vi "path_test.vi"() -> ()   [LabVIEW 2011]
panel:
  out "String":string
  out "size(s)":i32
  out "output string":string
  out "relative":bool
  out "array of strings":string[](array[string])
  in  "path 2":path
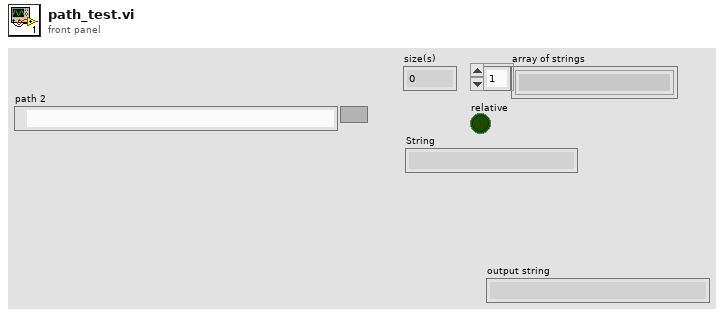
[diagram p1: front panel]
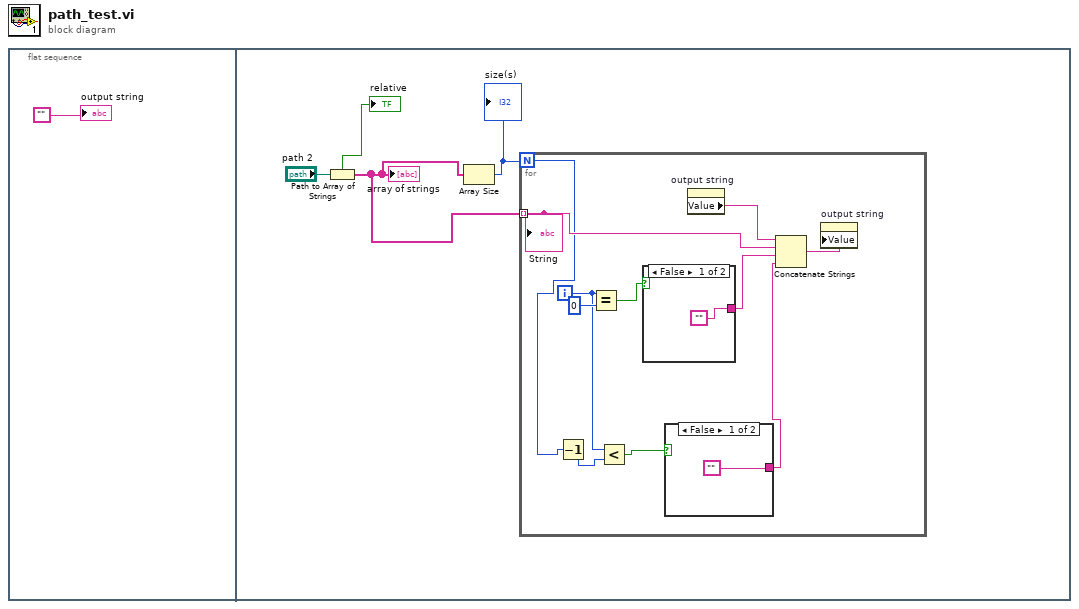
[diagram p0: block diagram]
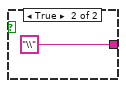
[diagram p2: hidden frame]
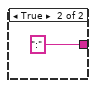
[diagram p3: hidden frame]
diagram:
  n1 = flat-sequence {
    frame #0 {
      "output string" <- ""
    }
    frame #1 {
      n2 = Path to Array of Strings(0:"path 2") -> (1:→"relative":bool, 2:w2:string[])
      "array of strings" <- w2
      n3 = Array Size(array=w2) -> (size(s)=w5:i32)
      "size(s)" <- w5
      n4 = for {
        N: w5 -> [w8]
        tunnel: w2 -> [w16] mode=indexing
        i -> [w10]
        n5 = Decrement(x=w8) -> (x-1=w7:i32)
        n6 = Equal?(x=w10, y=0) -> (x = y?=w12:bool)
        n7 = Less?(x=w10, y=w7) -> (x < y?=w9:bool)
        n8 = case shown="False" w12 {
          tunnel: ["" ":"] -> w11
          frame False {
          }
          frame True {
          }
        }
        n9 = case shown="False" w9 {
          tunnel: ["" "\\" ("string")] -> w6
          frame False {
          }
          frame True {
          }
        }
        n10 = property on="output string" class="Str"() -> ("Value"=w14:string)  [unwired: 2 in, 2 out]
        n11 = Concatenate Strings(w14, w16, w11, w6) -> (w15:string)
        n12 = property on="output string" class="Str"("Value"=w15) -> ()  [unwired: 2 in, 2 out]
        "String" <- w16
      }
    }
  }
